vi "PM100-Set Wavelength.vi"(0 "VISA in":refnum<visa-resource-name>, 7 "Lambda (nm)":dbl, 11 "error in (no error)":errorcluster) -> (4 "VISA out":refnum<visa-resource-name>, 15 "error out":errorcluster)   [LabVIEW 2015]
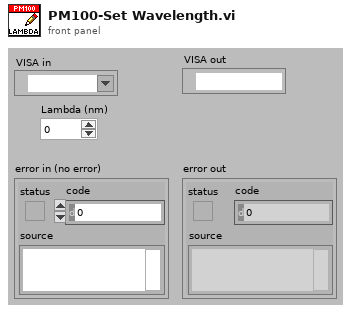
[diagram p1: front panel]
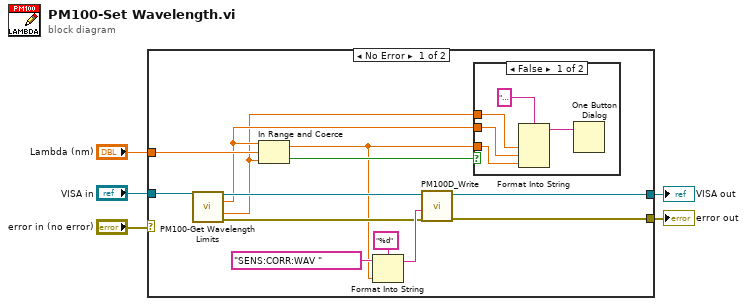
[diagram p0: block diagram]
diagram:
  n1 = case shown="No Error" "error in (no error)" {
    selector: "error in (no error)" -> [_ w25]
    tunnel: [w12 w25] -> w4
    tunnel: "VISA in" -> [w18 w24]
    tunnel: "Lambda (nm)" -> [w11 _]
    tunnel: [w6 w24] -> w1
    frame No Error {
      n2 = call "PM100-Get Wavelength Limits.vi"("VISA in"=w18) -> ("VISA out"=w17:refnum<visa-resource-name>, "WAV_MAX"=w8:dbl, "WAV_MIN"=w7:dbl, "error out"=w13:errorcluster)  [unwired: 10 in, 1 out]
      n3 = In Range and Coerce(upper limit=w8, x=w11, lower limit=w7) -> (coerced(x)=w9:dbl, In Range?=w10:bool)
      n4 = Format Into String(format string="%d", initial string="SENS:CORR:WAV " ("Command"), w9) -> (resulting string=w14:string)  [unwired: 1 in, 1 out]
      n5 = call "PM100D_Write.vi"("error in (no error)"=w13, "Command"=w14, "VISA in"=w17) -> ("error out"=w12:errorcluster, "VISA out"=w6:refnum<visa-resource-name>)  [unwired: 7 in]
      n6 = case shown="False" w10 {
        tunnel: w9 -> [w21 _]
        tunnel: w8 -> [w20 _]
        tunnel: w7 -> [w19 _]
        frame False {
          n7 = Format Into String(format string="Wavelength out of range for this power meter (%d - %dnm).\nMeter setting coerced to %d nm.", w19, w20, w21) -> (resulting string=w23:string)  [unwired: 2 in, 1 out]
          n8 = One Button Dialog(message=w23) -> ()  [unwired: 1 in, 1 out]
        }
        frame True {
        }
      }
    }
    frame Error {
    }
  }
  "error out" <- w4
  "VISA out" <- w1
